vi "object feature position.vi"(6 "Color":u32(colorbox)=65280, 8 "Error In":errorcluster, 10 "Feature Ponts":cluster{"X":sgl, "Y":sgl}[](array[cluster]), 11 "Image":T1) -> (0 "Error Out":errorcluster, 3 "Image Out":T1)   [LabVIEW 2014]
uses:
  <vilib>/vision/Image Controls.llb/IMAQ Image.ctl
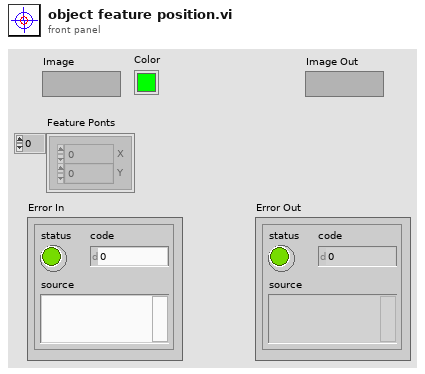
[diagram p1: front panel]
types:
  T1 = typedef "IMAQ Image.ctl" = refnum<image>
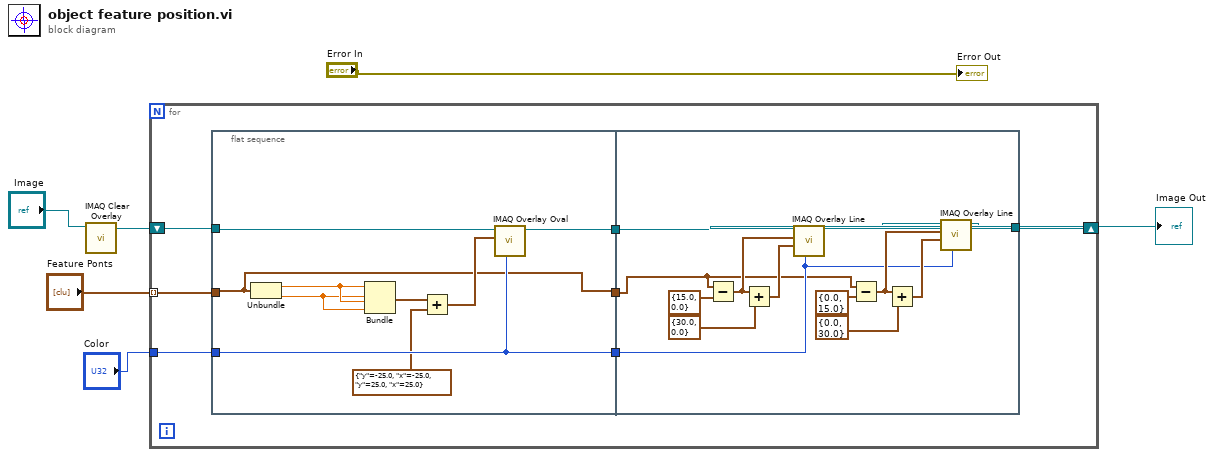
[diagram p0: block diagram]
diagram:
  n1 = call "IMAQ Clear Overlay"("Image"="Image") -> ("Image Out"=w4:T1)  [unwired: 2 in, 8 out]
  n2 = for {
    shift-right: [w11] -> w5
    shift-left: w4 -> [w13]
    tunnel: "Feature Ponts" -> [w10] mode=indexing
    tunnel: "Color" -> [w12]
    n3 = flat-sequence {
      tunnel: w10 -> [w14]
      tunnel: [w14] -> w9
      tunnel: w13 -> [w22]
      tunnel: w12 -> [w20]
      tunnel: [w20] -> w8
      tunnel: [w21] -> w7
      tunnel: w9 -> [w25]
      tunnel: w8 -> [w27]
      tunnel: [w24] -> w11
      tunnel: w7 -> [w23]
      frame #0 {
        n4 = Unbundle(w14) -> ("X"=w19:sgl, "Y"=w18:sgl)
        n5 = Bundle("X"=w19, "Y"=w18, "X"=w19, "Y"=w18) -> (w17:cluster{"X":sgl, "Y":sgl, "X":sgl, "Y":sgl})  [unwired: 1 out]
        n6 = Add(x=w17, y=cluster{"y":sgl, "x":sgl, "y":sgl, "x":sgl} {"y"=-25.0, "x"=-25.0, "y"=25.0, "x"=25.0}) -> (x+y=w15:cluster{sgl, sgl, sgl, sgl})
        n7 = call "IMAQ Overlay Oval"("Color"=w20, "Bounding Rectangle"=w15, "Image"=w22) -> ("Image Out"=w21:T1)  [unwired: 3 in, 5 out]
      }
      frame #1 {
        n8 = Subtract(x=w25, y=cluster{"x":sgl, "y":sgl} {"x"=15.0, "y"=0.0}) -> (x-y=w34:cluster{sgl, sgl})
        n9 = Add(x=w34, y=cluster{"x":sgl, "y":sgl} {"x"=30.0, "y"=0.0}) -> (x+y=w32:cluster{sgl, sgl})
        n10 = call "IMAQ Overlay Line"("Color"=w27, "End Point"=w32, "Start Point"=w34, "Image"=w23) -> ("Image Out"=w26:T1)  [unwired: 2 in, 5 out]
        n11 = Subtract(x=w25, y=cluster{"x":sgl, "y":sgl} {"x"=0.0, "y"=15.0}) -> (x-y=w30:cluster{sgl, sgl})
        n12 = Add(x=w30, y=cluster{"x":sgl, "y":sgl} {"x"=0.0, "y"=30.0}) -> (x+y=w31:cluster{sgl, sgl})
        n13 = call "IMAQ Overlay Line"("Color"=w27, "End Point"=w31, "Start Point"=w30, "Image"=w26) -> ("Image Out"=w24:T1)  [unwired: 2 in, 5 out]
      }
    }
  }
  "Image Out" <- w5
  "Error Out" <- "Error In"
